vi "Feed Immediate.vi"(7 "Description":string, 8 "Command Info In":T1, 9 "Deadband Value":dbl=0.01, 10 "Upper Setpoint":dbl, 11 "Lower Setpoint":dbl) -> (0 "Command Info Out":T1)   [LabVIEW 2019]
doc: "This template includes code for deadband comparision to avoid excessive command scheduling. It is particularly useful for joystick-driven commands.\n\nBe sure to right-click and select New from Template and save with a new command name."
uses:
  <vilib>/Rock Robotics/WPI/Framework/Command Status Info.ctl
  <vilib>/Rock Robotics/WPI/Framework/Completion Status.ctl
  <vilib>/Rock Robotics/WPI/Framework/Completion Notifier.ctl
  Implementation/Feed Setpoints.ctl
  Implementation/Feed Operations.ctl
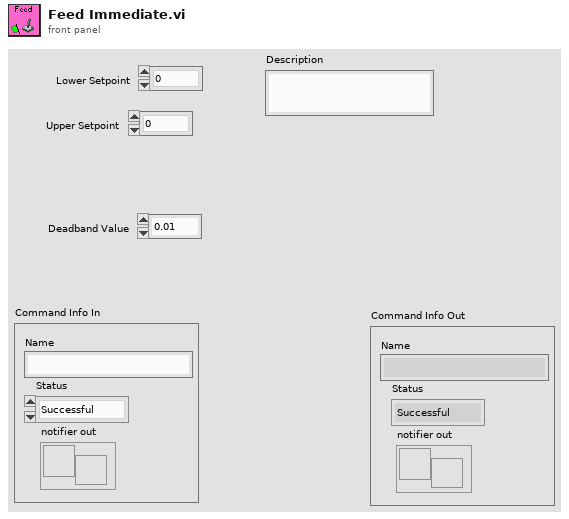
[diagram p1: front panel]
types:
  T1 = typedef "Command Status Info.ctl" = cluster{"Name":string, "Status":T2, "notifier out":T3}
  T2 = typedef "Completion Status.ctl" = enum16{"Successful", "Aborted", "Incomplete"}
  T3 = typedef "Completion Notifier.ctl" = refnum<notifier>
  T4 = typedef "Feed Setpoints.ctl" = cluster{"Operation":T5, "Lower Setpoint":dbl, "Upper Setpoint":dbl, "Duration":dbl}
  T5 = typedef "Feed Operations.ctl" = enum16{"Reserve", "Read Current", "Immediate", "Feed For Time"}
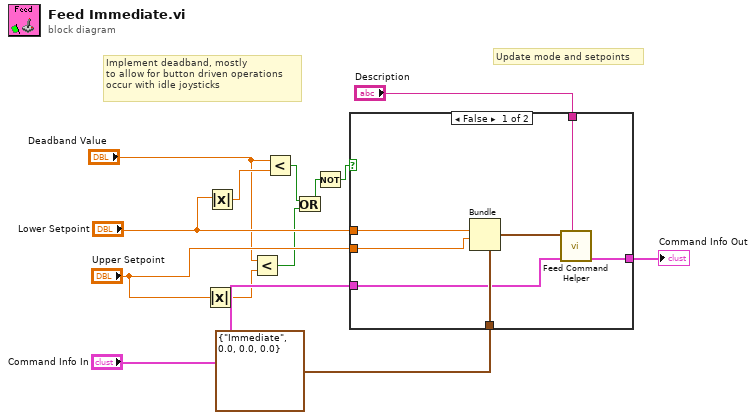
[diagram p0: block diagram]
diagram:
  # "Implement deadband, mostly\nto allow for button driven operations\noccur with idle joysticks"
  # "Update mode and setpoints"
  n1 = Absolute Value(x="Upper Setpoint") -> (abs(x)=w5:dbl)
  n2 = Absolute Value(x="Lower Setpoint") -> (abs(x)=w7:dbl)
  n3 = Less?(x="Deadband Value", y=w5) -> (x < y?=w3:bool)
  n4 = Less?(x="Deadband Value", y=w7) -> (x < y?=w4:bool)
  n5 = Or(x=w4, y=w3) -> (x .or. y?=w1:bool)
  n6 = Not(x=w1) -> (.not. x?=w2:bool)
  n7 = case shown="False" w2 {
    tunnel: "Lower Setpoint" -> [w20 _]
    tunnel: T4 {"Operation"=enum."Immediate", "Lower Setpoint"=0.0, "Upper Setpoint"=0.0, "Duration"=0.0} ("SubSystem Data") -> [w19 _]
    tunnel: [w18 w21] -> w13
    tunnel: "Command Info In" -> [w17 w21]
    tunnel: "Description" -> [w15 _]
    tunnel: "Upper Setpoint" -> [w14 _]
    frame False {
      n8 = Bundle(cluster=w19, "Lower Setpoint"=w20, "Upper Setpoint"=w14) -> (w16:T4)  [unwired: 2 in]
      n9 = call "Feed Command Helper.vi"("Description"=w15, "Command Info In"=w17, "SubSystem Data"=w16) -> ("Command Info Out"=w18:T1)  [unwired: 6 in, 2 out]
    }
    frame True {
    }
  }
  "Command Info Out" <- w13
